vi "Editor.vi"() -> ()   [LabVIEW 2020]
uses:
  TypeDef/display.ctl
  TypeDef/tiles.ctl
panel:
  out "size(s)":i32[](array[numeric])
  in  "stop":bool
  in  "Display":T1
  in  "Size":i32
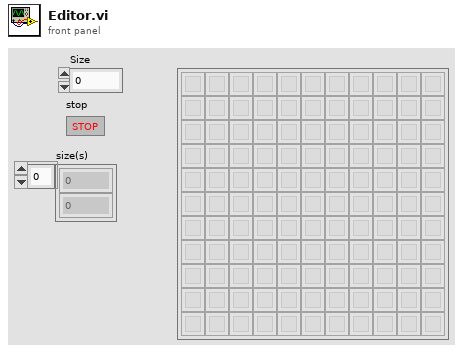
[diagram p1: front panel]
types:
  T1 = typedef "display.ctl" = T2[][]
  T2 = typedef "tiles.ctl" = u16
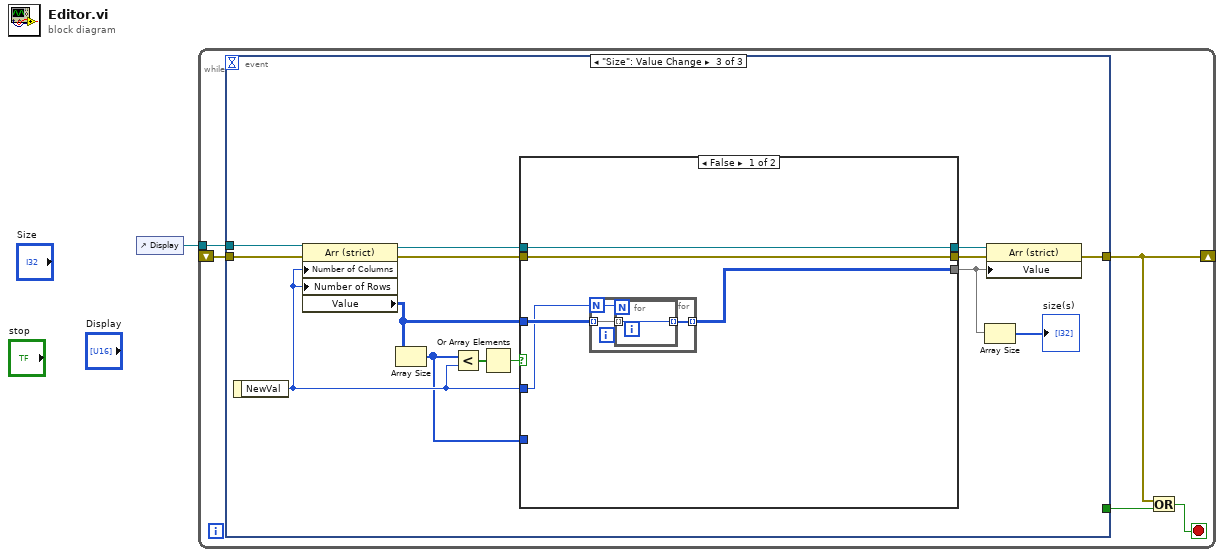
[diagram p0: block diagram]
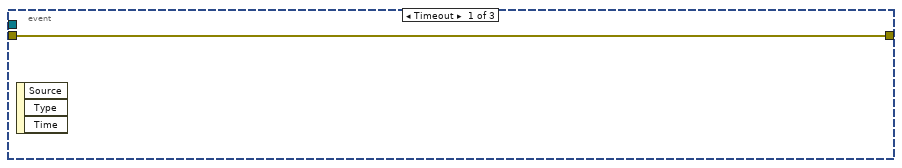
[diagram p2: hidden frame]
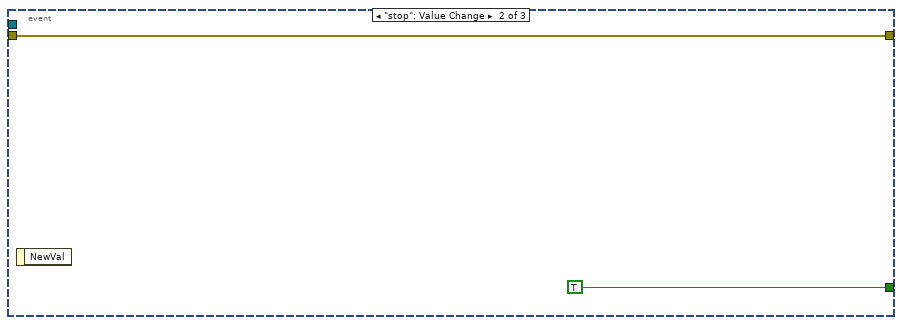
[diagram p3: hidden frame]
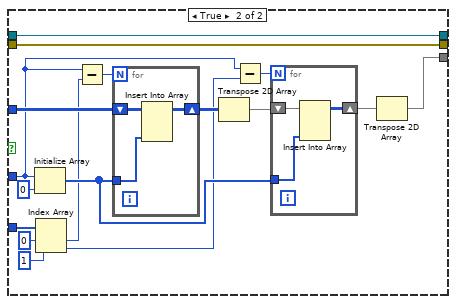
[diagram p4: hidden frame]
diagram:
  n1 = control-ref of="Display"() -> (w1:refnum<vi>)
  n2 = while {
    shift-right: [w4] -> _
    shift-left: _ -> [w6]
    tunnel: w1 -> [w2]
    stop <- w5 stop-if-true
    n3 = event shown="[2] \"Size\": Value Change" {
      selector: _ -> [_ _ _]
      dyn-events: _ -> [_ _ _]
      timeout: _ -> [_ _ _]
      tunnel: [_ TRUE _] -> w3
      tunnel: w6 -> [w7 w8 w23]
      tunnel: [w7 w8 w17] -> w4
      tunnel: w2 -> [_ _ w10]
      event Timeout {
        n4 = event-data() -> ()  [unwired: 1 in, 3 out]
      }
      event "stop": Value Change {
        n5 = event-data() -> ()  [unwired: 1 in, 1 out]
      }
      event "Size": Value Change {
        n6 = event-data() -> ("NewVal"=w18:i32)  [unwired: 1 in]
        n7 = property class="Arr (strict)"(reference=w10, error in=w23, "Number of Columns"=w18, "Number of Rows"=w18) -> (reference out=w15:refnum<vi>, error out=w21:errorcluster, "Value"=w20:T1)
        n8 = Array Size(array=w20) -> (size(s)=w11:i32[])
        n9 = Less?(x=w11, y=w18) -> (x < y?=w22:bool[])
        n10 = Or Array Elements(Boolean array=w22) -> (logical OR=w19:bool)
        n11 = case shown="False" w19 {
          tunnel: w21 -> [w28 w39]
          tunnel: [w28 w39] -> w16
          tunnel: w20 -> [w26 w47]
          tunnel: w18 -> [w24 w41]
          tunnel: [w25 w40] -> w13
          tunnel: w15 -> [w27 w38]
          tunnel: [w27 w38] -> w14
          tunnel: w11 -> [_ w37]
          frame False {
            n12 = for {
              N: w24 -> [w29]
              tunnel: w26 -> [w31] mode=indexing
              tunnel: [w30] -> w25 mode=indexing
              n13 = for {
                N: w29 -> [_]
                tunnel: w31 -> [w32] mode=indexing
                tunnel: [w32] -> w30 mode=indexing
              }
            }
          }
          frame True {
            n14 = Initialize Array(w41, 0 ("dimension size")) -> (w42:i32[])
            n15 = Index Array(array=w37, index #1=0 ("index"), index #2=1 ("index")) -> (element #1=w34:i32, element #2=w33:i32)
            n16 = Subtract(x=w41, y=w34) -> (x-y=w48:i32)
            n17 = for {
              N: w48 -> [_]
              tunnel: w42 -> [w54]
              shift-right: [w53] -> w46
              shift-left: w47 -> [w55]
              n18 = Insert Into Array(array=w55, new element=w54) -> (w53:T1)  [unwired: 2 in]
            }
            n19 = Transpose 2D Array(2D array=w46) -> (transposed array=w43:T1)
            n20 = Subtract(x=w41, y=w33) -> (x-y=w45:i32)
            n21 = for {
              N: w45 -> [_]
              tunnel: w42 -> [w51]
              shift-right: [w50] -> w44
              shift-left: w43 -> [w52]
              n22 = Insert Into Array(array=w52, new element=w51) -> (w50:T1)  [unwired: 2 in]
            }
            n23 = Transpose 2D Array(2D array=w44) -> (transposed array=w40:T1)
          }
        }
        n24 = Array Size(array=w13) -> (size(s)=→"size(s)":i32[])
        n25 = property class="Arr (strict)"(reference=w14, error in=w16, "Value"=w13) -> (error out=w17:errorcluster)  [unwired: 1 out]
      }
    }
    n26 = Or(x=w4, y=w3) -> (x .or. y?=w5:bool)
  }
